vi "4Pi 4Pi Modes - Astig Modes AE.vi"(0 "Coefficients In":cluster{"Mode":string, "Amplitude":dbl}[](array[cluster]), 2 "Action":T1, 5 "Enabled In":bool=TRUE) -> (4 "Coefficients Out":cluster{"Mode":string, "Amplitude":dbl}[](array[cluster]), 6 "Enabled Out":bool)   [LabVIEW 2016]
uses:
  Hardware Configuration/Hardware Configuration Controls/Standard Action.ctl
panel:
  out "Zerored Value":cluster{"Mode":string, "Amplitude":dbl}[](array[cluster])
  out "Stored Value":cluster{"Mode":string, "Amplitude":dbl}[](array[cluster])
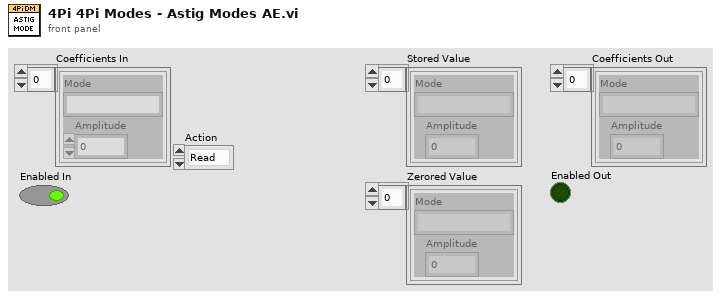
[diagram p1: front panel]
types:
  T1 = typedef "Standard Action.ctl" = enum16{"Read", "Write"}
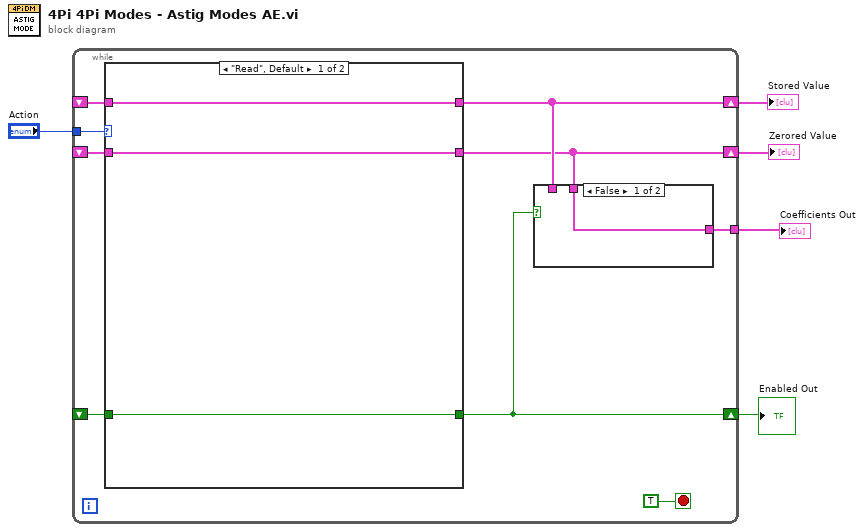
[diagram p0: block diagram]
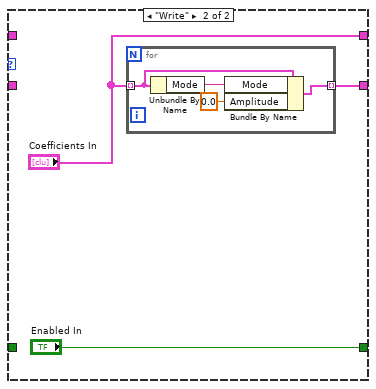
[diagram p3: hidden frame]
diagram:
  n1 = while {
    tunnel: "Action" -> [w14]
    shift-right: [w11] -> w4
    shift-left: _ -> [w12]
    shift-right: [w10] -> w3
    shift-left: _ -> [w8]
    shift-right: [w9] -> w2
    shift-left: _ -> [w7]
    tunnel: [w6] -> w1
    stop <- TRUE stop-if-true
    n2 = case shown="\"Read\", Default" w14 {
      tunnel: w12 -> [w19 _]
      tunnel: [w19 "Enabled In"] -> w11
      tunnel: [w17 w21] -> w9
      tunnel: [w18 "Coefficients In"] -> w10
      tunnel: w8 -> [w18 _]
      tunnel: w7 -> [w17 _]
      frame "Read", Default {
      }
      frame "Write" {
        n3 = for {
          tunnel: "Coefficients In" -> [w25] mode=indexing
          tunnel: [w23] -> w21 mode=indexing
          n4 = Unbundle By Name(w25) -> ("Mode"=w26:string)
          n5 = Bundle By Name(cluster=w25, "Mode"=w26, "Amplitude"=0.0) -> (w23:cluster{"Mode":string, "Amplitude":dbl})
        }
      }
    }
    n6 = case shown="False" w11 {
      tunnel: w10 -> [_ w16]
      tunnel: w9 -> [w15 _]
      tunnel: [w15 w16] -> w6
      frame False {
      }
      frame True {
      }
    }
  }
  "Coefficients Out" <- w1
  "Enabled Out" <- w4
  "Stored Value" <- w3
  "Zerored Value" <- w2
